vi "rqcBob Error Handler.vi"(8 "error in (no error)":errorcluster, 11 "rqcBob ServiceNET control":T1) -> (0 "error out":errorcluster, 2 "error sequence":T2[](array[typedef]))   [LabVIEW 2018]
uses:
  Custom Controls/rqcBob States.ctl
  Shared/Shared Host Lib/rqc ServiceNET/Bob/Custom Controls/rqcBob ServiceNET control.ctl
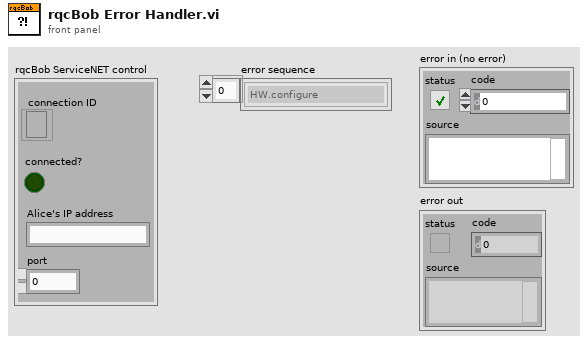
[diagram p1: front panel]
types:
  T1 = typedef "rqcBob ServiceNET control.ctl" = cluster{"connection ID":refnum<k5>, "connected?":bool, "Alice's IP address":string, "port":u16}
  T2 = typedef "rqcBob States.ctl" = enum16{"HW.configure", "HW.sendTrigger", "HW.initiate", "HW.measure", "HW.stop", "NET.create", "NET.connect", "NET.sendCommand", "NET.readCommand", "NET.readData", "NET.close", "App.HandleEvent", "App.HandleError", "App.Stop"}
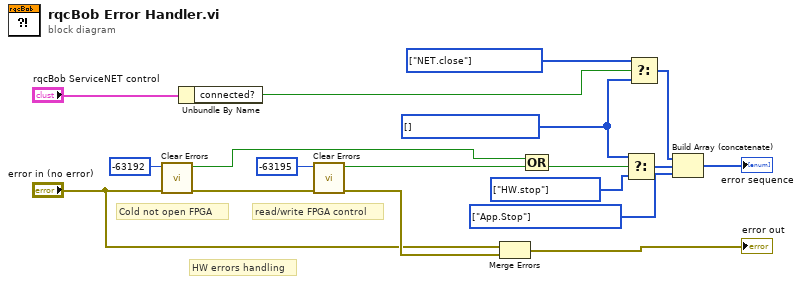
[diagram p0: block diagram]
diagram:
  w14 = T2[] [enum."HW.stop"] items=["HW.configure", "HW.sendTrigger", "HW.initiate", "HW.measure", "HW.stop", "NET.create", "NET.connect", "NET.sendCommand", "NET.readCommand", "NET.readData", "NET.close", "App.HandleEvent", "App.HandleError", "App.Stop"]
  w15 = T2[] [] items=["HW.configure", "HW.sendTrigger", "HW.initiate", "HW.measure", "HW.stop", "NET.create", "NET.connect", "NET.sendCommand", "NET.readCommand", "NET.readData", "NET.close", "App.HandleEvent", "App.HandleError", "App.Stop"]
  w11 = T2[] [enum."NET.close"] items=["HW.configure", "HW.sendTrigger", "HW.initiate", "HW.measure", "HW.stop", "NET.create", "NET.connect", "NET.sendCommand", "NET.readCommand", "NET.readData", "NET.close", "App.HandleEvent", "App.HandleError", "App.Stop"]
  w17 = T2[] [enum."App.Stop"] items=["HW.configure", "HW.sendTrigger", "HW.initiate", "HW.measure", "HW.stop", "NET.create", "NET.connect", "NET.sendCommand", "NET.readCommand", "NET.readData", "NET.close", "App.HandleEvent", "App.HandleError", "App.Stop"]
  # "HW errors handling"
  # "Cold not open FPGA"
  # "read/write FPGA control"
  n1 = call <vilib>:"Clear Errors.vi"("error in (no error)"="error in (no error)", "specific error code to clear (0: all)"=-63192) -> ("error out"=w6:errorcluster, "specific error cleared?"=w4:bool)  [unwired: 4 in]
  n2 = Unbundle By Name("rqcBob ServiceNET control") -> ("connected?"=w10:bool)
  n3 = call <vilib>:"Clear Errors.vi"("error in (no error)"=w6, "specific error code to clear (0: all)"=-63195) -> ("error out"=w2:errorcluster, "specific error cleared?"=w13:bool)  [unwired: 4 in]
  n4 = Merge Errors("error in (no error)", w2) -> (→"error out":errorcluster)
  n5 = Compound Arithmetic op=OR(w4, w13) -> (w5:bool)
  n6 = Select(t=w15, s=w5, f=w14) -> (s? t:f=w16:T2[])
  n7 = Select(t=w11, s=w10, f=w15) -> (s? t:f=w12:T2[])
  n8 = Build Array (concatenate)(w12, w16, w17) -> (→"error sequence":T2[])
